vi "Excel_data.vi"() -> (1 "i_Data":i32, 2 "Data":cluster{dbl, dbl, dbl, dbl}(graph))   [LabVIEW 2011]
uses:
  <vilib>/Utility/file.llb/Read From Spreadsheet File (DBL).vi
panel:
  out "element":dbl
  out "Vex":dbl format="%#.2f"
  out "File patch":path
  out "Iex":dbl format="%#.2f"
  out "Gex":dbl format="%#.2f"
  in  "stop":bool
  out "Tex":dbl format="%#.2f"
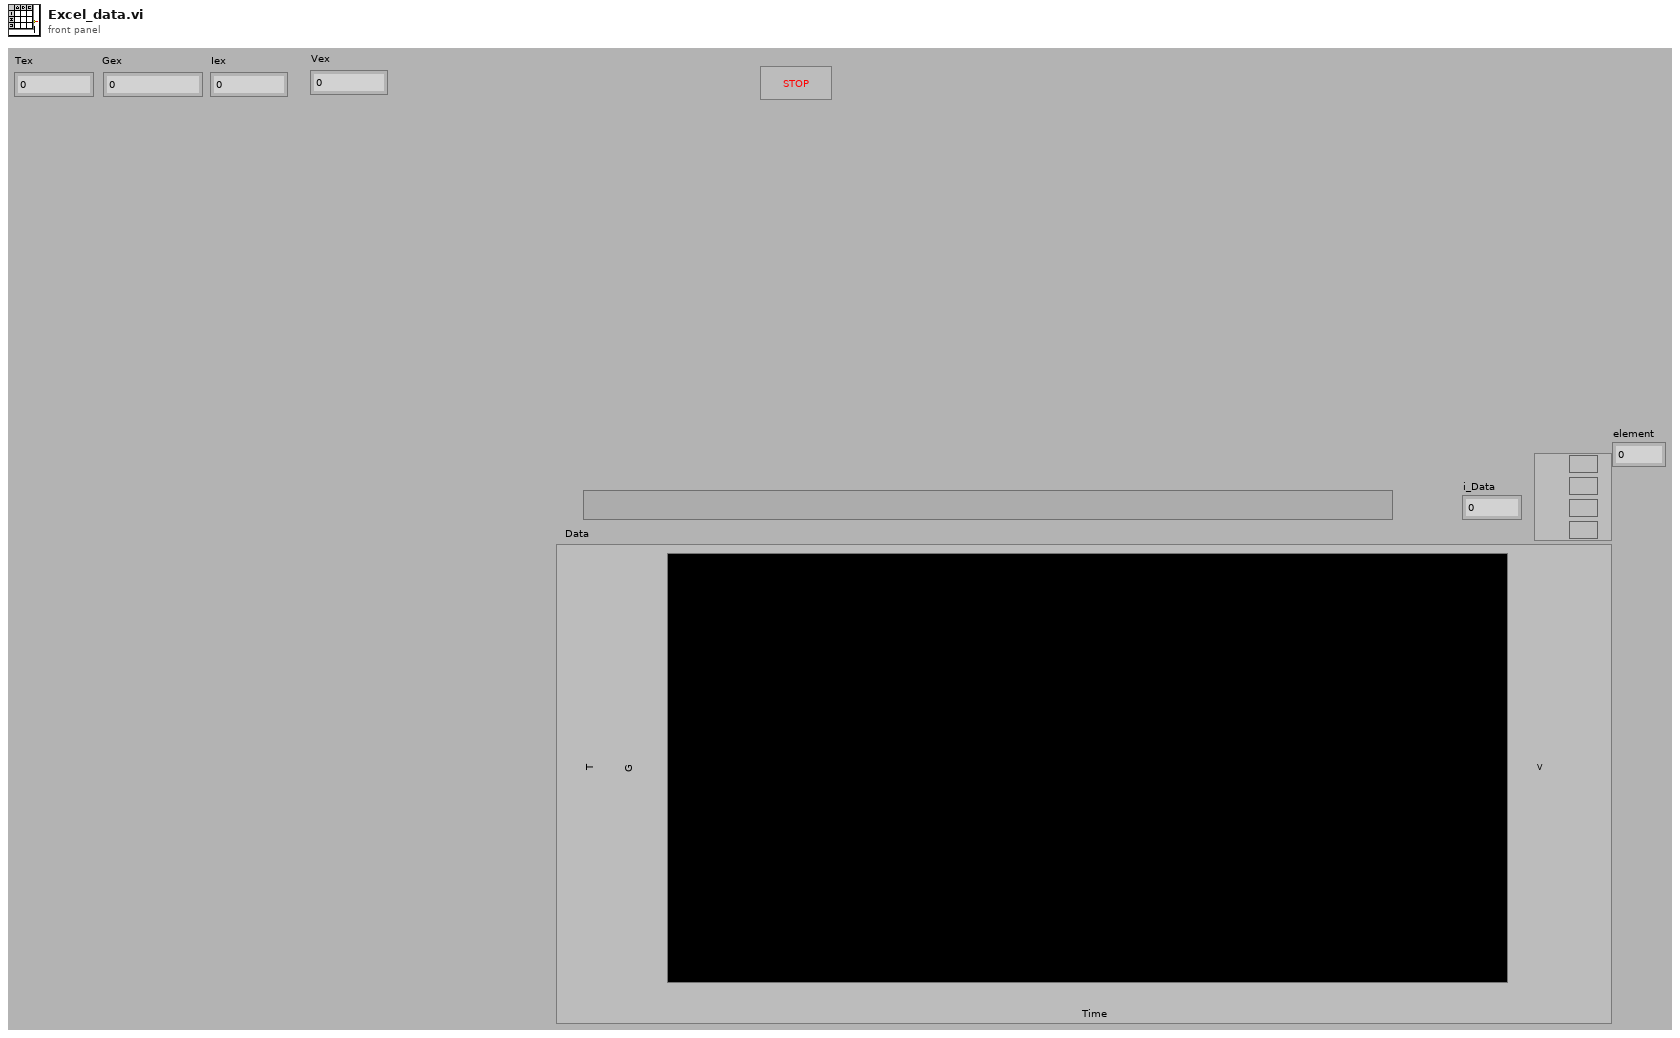
[diagram p1: front panel]
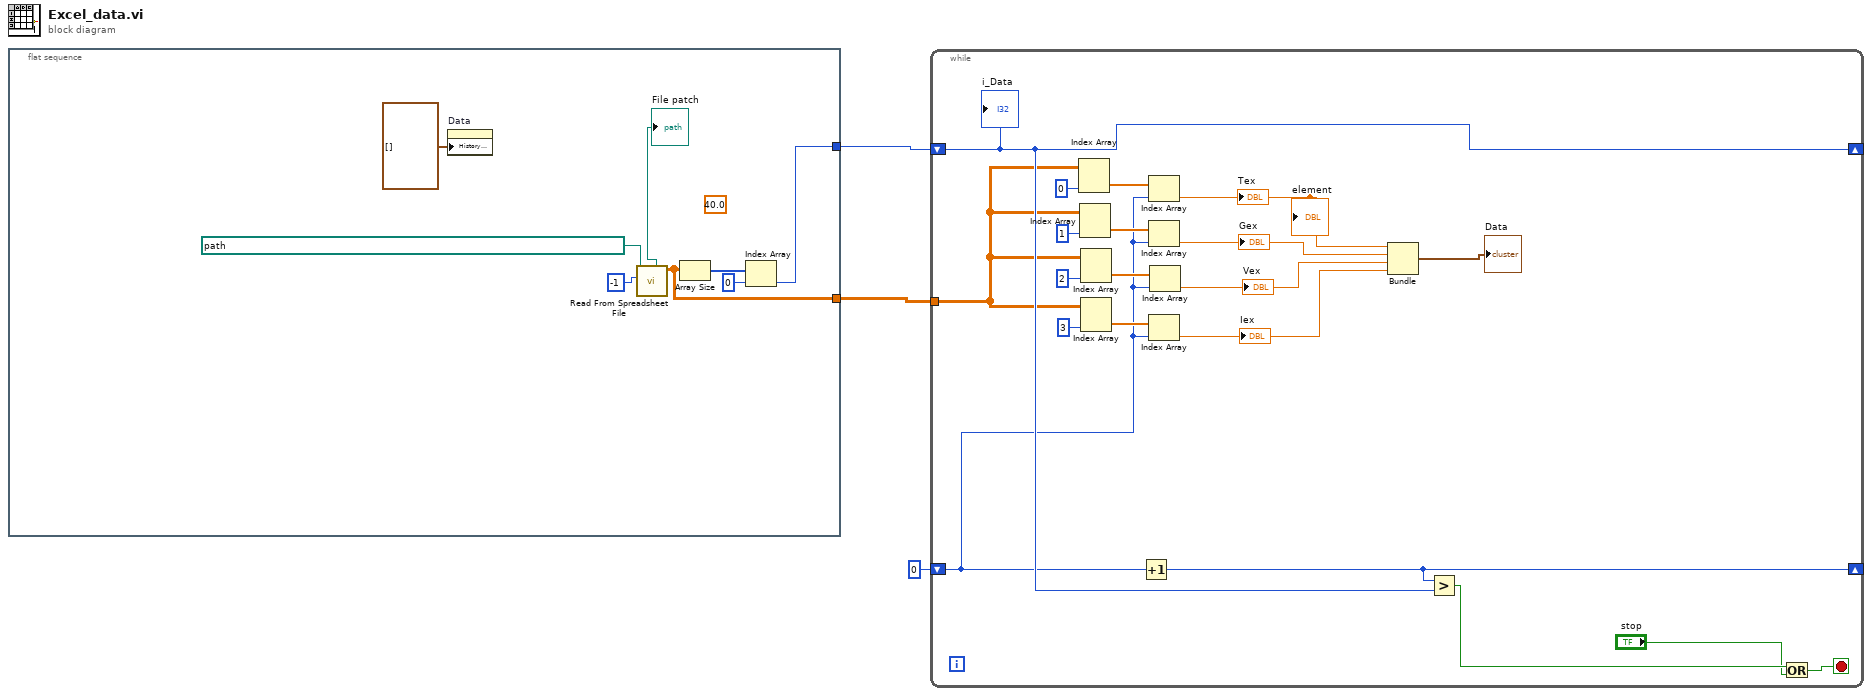
[diagram p0: block diagram]
diagram:
  n1 = flat-sequence {
    tunnel: [w7] -> w1
    tunnel: [w8] -> w3
    frame #0 {
      (unwired) 40.0 ("Derinlik")
      n2 = property on="Data" class="WFChart (strict)"("History Data"=cluster{dbl, dbl, dbl, dbl}[] []) -> ()  [unwired: 2 in, 2 out]
      n3 = call-poly <vilib>:"Read From Spreadsheet File.vi"("number of rows (all:-1)"=-1, "file path (dialog if empty)"=path "D:/YüksekLisans/Tez/uygula/LabView Program/Suleyman_TEZ/sadePanel1.xls") -> ("all rows"=w8:dbl[][], "new file path (Not A Path if cancelled)"=→"File patch":path)  [unwired: 2 in, 6 out]
      n4 = Array Size(array=w8) -> (size(s)=w9:i32[])
      n5 = Index Array(array=w9, index=0 ("index 2")) -> (element=w7:i32)
    }
  }
  n6 = while {
    tunnel: w3 -> [w17]
    shift-right: [w21] -> _
    shift-left: w1 -> [w21]
    shift-right: [w23] -> _
    shift-left: 0 -> [w18]
    stop <- w20 stop-if-true
    n7 = Index Array(array=w17, index (col)=0 ("disabled index (col)")) -> (element=w27:dbl[])  [unwired: 1 in]
    n8 = Index Array(array=w17, index (col)=1 ("disabled index (col)")) -> (element=w24:dbl[])  [unwired: 1 in]
    n9 = Index Array(array=w17, index (col)=2 ("disabled index (col)")) -> (element=w25:dbl[])  [unwired: 1 in]
    n10 = Index Array(array=w17, index (col)=3 ("disabled index (col)")) -> (element=w26:dbl[])  [unwired: 1 in]
    n11 = Increment(x=w18) -> (x+1=w23:i32)
    n12 = Index Array(array=w27, index=w18) -> (element=w16:dbl)
    "Tex" <- w16
    "element" <- w16
    n13 = Index Array(array=w24, index=w18) -> (element=w13:dbl)
    "Gex" <- w13
    n14 = Index Array(array=w26, index=w18) -> (element=w14:dbl)
    "Iex" <- w14
    n15 = Index Array(array=w25, index=w18) -> (element=w15:dbl)
    "Vex" <- w15
    n16 = Bundle(w16, w13, w15, w14) -> (→"Data":cluster{dbl, dbl, dbl, dbl})  [unwired: 1 out]
    n17 = Greater?(x=w23, y=w21) -> (0:w22:bool)
    n18 = Or(x=w22, y="stop") -> (x .or. y?=w20:bool)
    "i_Data" <- w21
  }
